vi "Profile C Generation v1.vi"() -> ()   [LabVIEW 2018]
uses:
  <vilib>/Utility/file.llb/Write Delimited Spreadsheet (DBL).vi
  <vilib>/express/express analysis/Spectral/Block/exnSpectralBlock spectral measurements power poly.vi
  <vilib>/express/express analysis/Spectral/Block/exnSpectralBlock spectral measurements power WFM.vi
  <vilib>/addons/Time Series Analysis/Statistical Analysis.llb/TSA Normal Distribution Test (Array).vi
  <vilib>/express/express analysis/Spectral/XNode/ExpressSpectralMeasurementsBlockNode.xnode
  <vilib>/addons/_Advanced Signal Processing/NI_AdvSigProcTSA.lvlib
  <vilib>/measure/NI_MABase.lvlib
panel:
  in  "Ramp multiplier":dbl=20.0 format="%#_13g"
  in  "Dwell multiplier":dbl=20.0 format="%#_13g"
  in  "filter specifications":T1={"lower cutoff freq"=0.1, "higher cutoff freq"=2.0, "order"=5}
  in  "Standard Deviation":dbl=0.0009148153893115104
  in  "exponent 2":dbl=0.8 format="%.2p"
  in  "noise density":dbl=0.47 format="%.2p"
  out "Power Spectrum (Hanning window)":cluster{"f0":dbl, "df":dbl, "magnitude":dbl[]}(graph)
  out "Histogram":cluster{"Axis":dbl[], dbl[]}[](graph)
  out "Data":dbl[][](graph)
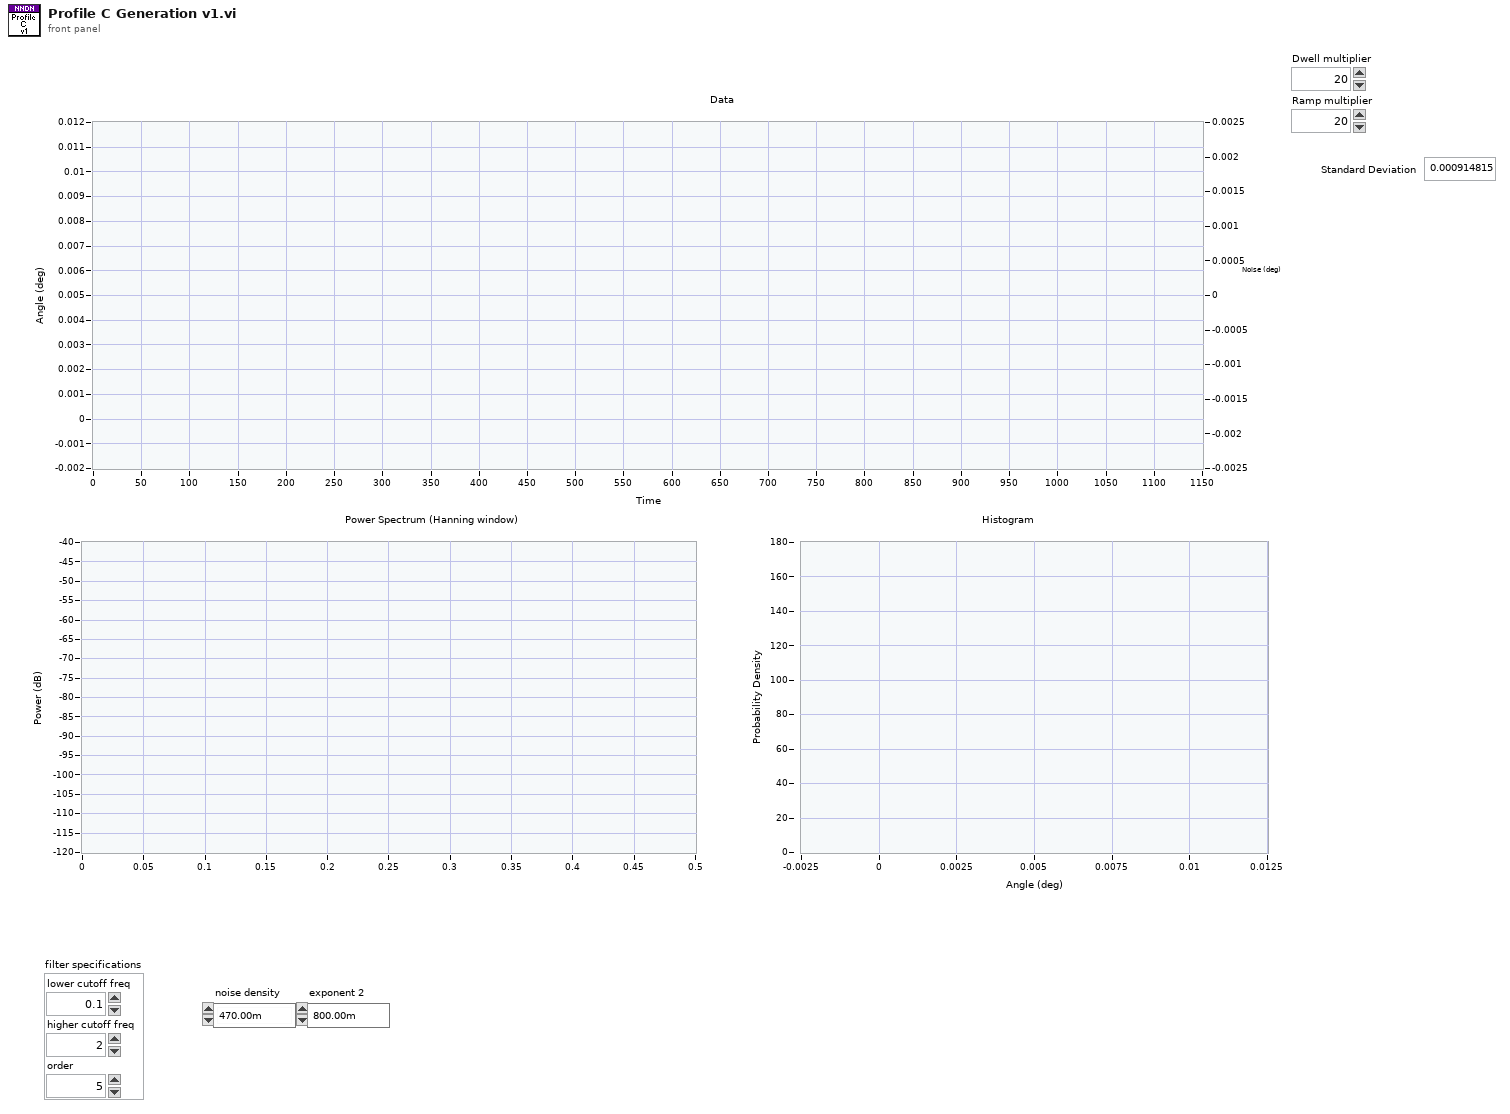
[diagram p1: front panel]
types:
  T1 = cluster{"lower cutoff freq":dbl, "higher cutoff freq":dbl, "order":i32}
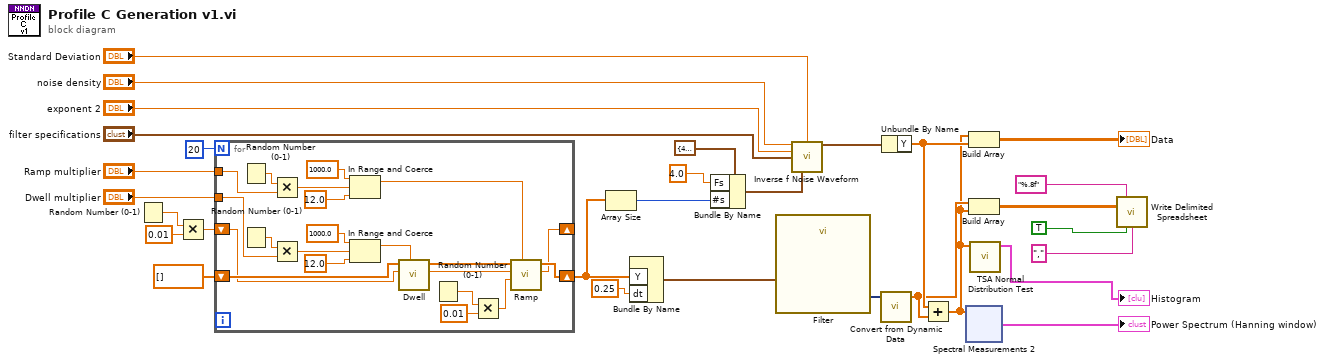
[diagram p0: block diagram]
diagram:
  n1 = Random Number (0-1)() -> (number: 0 to 1=w10:dbl)
  n2 = Multiply(x=w10, y=0.01) -> (x*y=w8:dbl)
  n3 = for {
    N: 20 -> [_]
    tunnel: "Dwell multiplier" -> [w50]
    shift-right: [w32] -> w6
    shift-left: dbl[] [] ("Array Out") -> [w49]
    tunnel: "Ramp multiplier" -> [w42]
    shift-right: [w31] -> _
    shift-left: w8 -> [w33]
    n4 = Random Number (0-1)() -> (number: 0 to 1=w43:dbl)
    n5 = Random Number (0-1)() -> (number: 0 to 1=w51:dbl)
    n6 = Multiply(x=w43, y=w42) -> (x*y=w37:dbl)
    n7 = Multiply(x=w51, y=w50) -> (x*y=w41:dbl)
    n8 = In Range and Coerce(upper limit=1000.0, x=w37, lower limit=12.0) -> (coerced(x)=w34:dbl)  [unwired: 1 out]
    n9 = In Range and Coerce(upper limit=1000.0, x=w41, lower limit=12.0) -> (coerced(x)=w40:dbl)  [unwired: 1 out]
    n10 = call "Dwell.vi"("Points"=w40, "Angle"=w33, "Array In"=w49) -> ("Last Point"=w47:dbl, "Array Out"=w48:dbl[])  [unwired: 7 in]
    n11 = Random Number (0-1)() -> (number: 0 to 1=w45:dbl)
    n12 = Multiply(x=w45, y=0.01) -> (x*y=w44:dbl)
    n13 = call "Ramp.vi"("Points"=w34, "End Angle"=w44, "Start Angle"=w47, "Array In"=w48) -> ("Last Value"=w31:dbl, "Array Out"=w32:dbl[])  [unwired: 6 in]
  }
  n14 = Array Size(array=w6) -> (size(s)=w14:i32)
  n15 = Bundle By Name("Y"=w6, "dt"=0.25) -> (w5:waveform(dbl))  [unwired: 1 in]
  n16 = Bundle By Name(cluster=cluster{"Fs":dbl, "#s":dbl} {"Fs"=4.0, "#s"=1000.0} ("sampling info"), "Fs"=4.0, "#s"=w14) -> (w19:cluster{"Fs":dbl, "#s":dbl})
  n17 = call "Filter"("Signal"=w5) -> ("Filtered Signal"=w7:dynamicdata)  [unwired: 9 in, 1 out]
  n18 = call <vilib>:"Inverse f Noise Waveform.vi"("noise density"="noise density", "standard deviation"="Standard Deviation", "exponent"="exponent 2", "filter specifications"="filter specifications", "sampling info"=w19) -> ("signal out"=w21:waveform(dbl))  [unwired: 6 in, 4 out]
  n19 = call "Convert from Dynamic Data"("Dynamic Data Type"=w7) -> ("Array"=w3:dbl[])  [unwired: 3 in]
  n20 = Unbundle By Name(w21) -> ("Y"=w15:dbl[])
  n21 = Add(x=w15, y=w3) -> (x+y=w1:dbl[])
  n22 = xnode "Spectral Measurements 2"("Signals"=w1) -> ("Power Spectrum"=→"Power Spectrum (Hanning window)":cluster{"f0":dbl, "df":dbl, "magnitude":dbl[]})  [unwired: 1 in, 1 out]
  n23 = Build Array(w1, w15) -> (→"Data":dbl[][])
  n24 = Build Array(w3, w1) -> (w16:dbl[][])
  n25 = call-poly <vilib>:"TSA Normal Distribution Test.vi"("Xt"=w1) -> ("histogram"=→"Histogram":cluster{"Axis":dbl[], dbl[]}[])  [unwired: 9 in, 1 out]
  n26 = call-poly <vilib>:"Write Delimited Spreadsheet.vi"("format (%.3f)"="%.8f", "2D data"=w16, "transpose? (no:F)"=TRUE, "delimiter (\\t)"="," ("delimiter (\\t)")) -> ()  [unwired: 10 in, 2 out]
